vi "libssh2_channel_exec.vi"(8 "error in (no error)":errorcluster, 10 "command":string, 11 "channel":T1) -> (0 "error out":errorcluster)   [LabVIEW 2017, in "libssh2.lvlib"]
doc: "Execute a command on the SSH server."
uses:
  libssh2.lvlib
  Channel Refnum.ctl
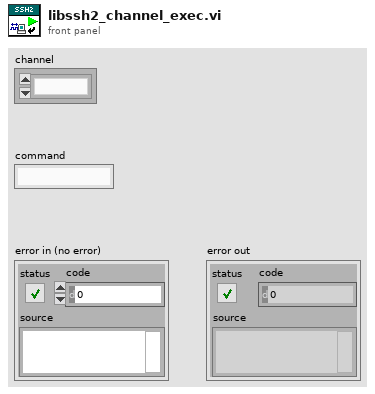
[diagram p1: front panel]
types:
  T1 = typedef "libssh2.lvlib/Channel Refnum.ctl" = refnum<k1>
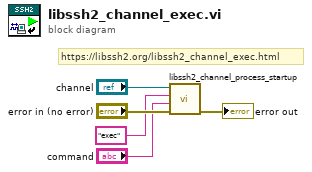
[diagram p0: block diagram]
diagram:
  # "https://libssh2.org/libssh2_channel_exec.html"
  n1 = call "libssh2_channel_process_startup.vi"("error in (no error)"="error in (no error)", "message"="command", "request"="exec", "channel"="channel") -> ("error out"=→"error out":errorcluster)  [unwired: 7 in]
